vi "Lab_Temp_PID.vi"(1 "Present Value":dbl=15.0 format="%.2f", 2 "Previous Control Sum":dbl format="%.2f", 3 "Setpoint":dbl=15.0 format="%.2f") -> (0 "Dem Output":dbl format="%.2f")   [LabVIEW 2011]
uses:
  <vilib>/Analysis/NI_AALPro.lvlib
panel:
  in  "O/P deadband":dbl=0.5 format="%.2f"
  in  "Kp Deadband":dbl format="%.2f"
  in  "Derivative History":i32=20
  out "deadbanded error":dbl format="%.2f"
  in  "P":bool=TRUE
  in  "D":bool=TRUE
  in  "I":bool=TRUE
  out "Waveform Chart":T1(graph)
  in  "Manual Demand":dbl min=0.0 max=100.0 format="%.2f"
  in  "Manual Override":bool
  out "Control Sum":dbl format="%.2f"
  out "Derivative Term":dbl format="%.2f"
  out "Integral Term":dbl format="%.2f"
  out "error differential":dbl format="%.5f"
  out "error integral":dbl format="%.2f"
  out "Proportional Term":dbl format="%.2f"
  in  "Kd":dbl=50.0 format="%.2f"
  in  "Ki":dbl=40.0 format="%.2f"
  in  "Kp":dbl=30.0 format="%.2f"
  out "error":dbl format="%.2f"
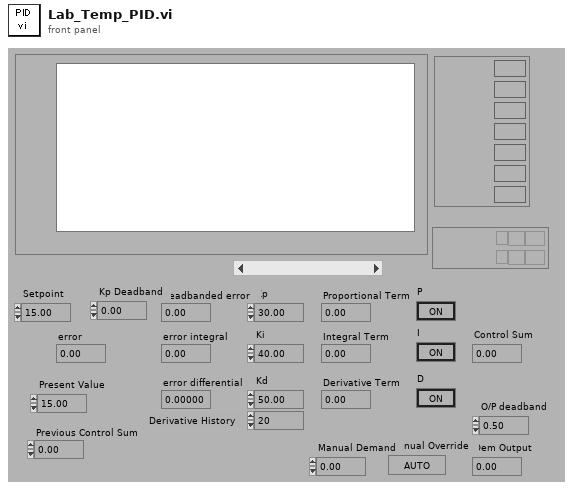
[diagram p1: front panel]
types:
  T1 = cluster{"Setpoint":dbl, "Present Value":dbl, "Proportional Term":dbl, "Integral Term":dbl, "Derivative Term":dbl, "Control Sum":dbl, "Dem Output":dbl}
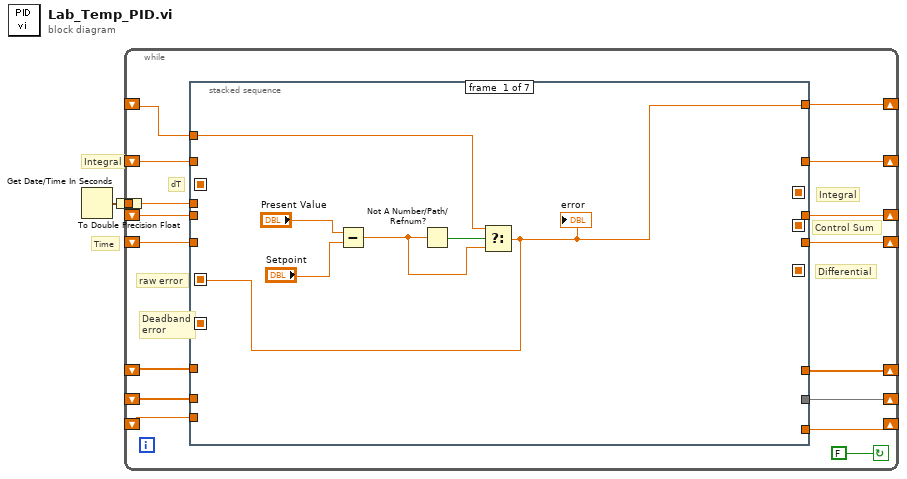
[diagram p0: block diagram]
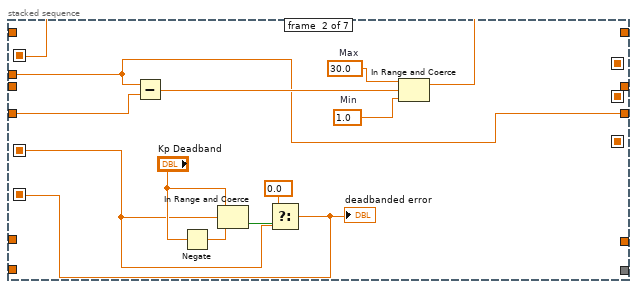
[diagram p2: hidden frame]
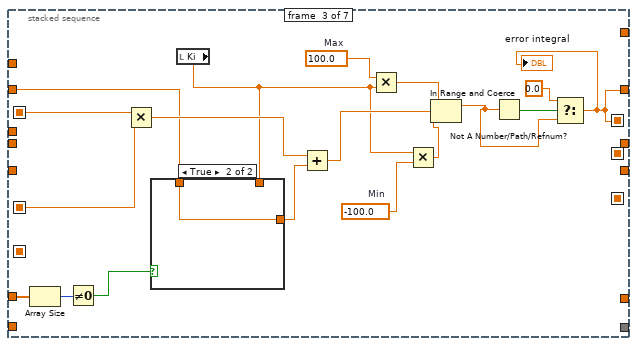
[diagram p3: hidden frame]
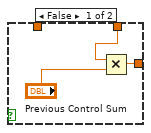
[diagram p4: hidden frame]
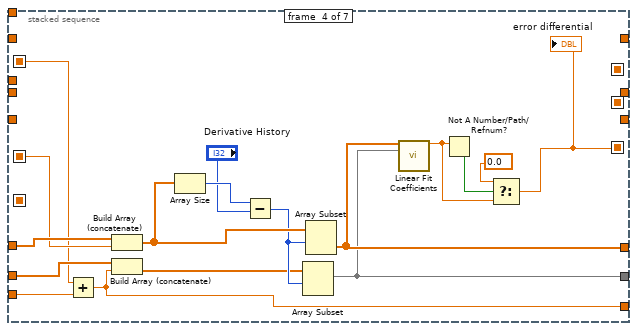
[diagram p5: hidden frame]
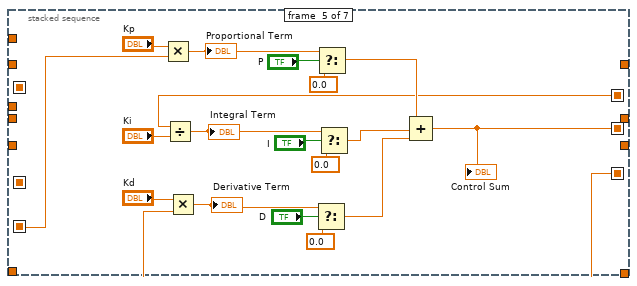
[diagram p6: hidden frame]
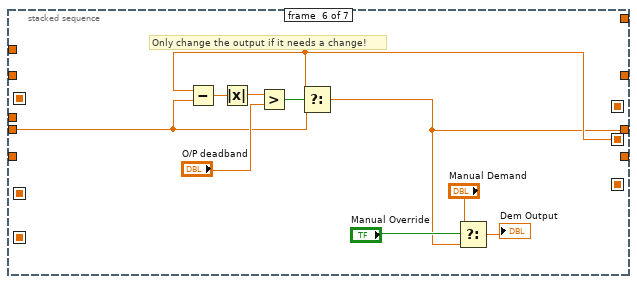
[diagram p7: hidden frame]
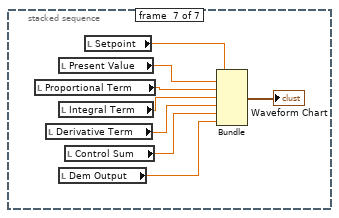
[diagram p8: hidden frame]
diagram:
  # "Integral"
  # "Time"
  n1 = Get Date/Time In Seconds() -> (seconds since 1Jan1904=w1:timestamp)
  n2 = To Double Precision Float(number=w1) -> (double precision float=w2:dbl)
  n3 = while {
    shift-left: _ -> [w5]
    shift-right: [w4] -> _
    shift-left: _ -> [w7]
    shift-right: [w6] -> _
    shift-left: _ -> [w9]
    shift-right: [w8] -> _
    tunnel: w2 -> [w14]
    shift-left: _ -> [w11]
    shift-right: [w10] -> _
    shift-left: _ -> [w13]
    shift-right: [w12] -> _
    shift-left: _ -> [w15]
    shift-right: [w16] -> _
    shift-left: _ -> [w18]
    shift-right: [w17] -> _
    stop <- FALSE continue-if-true
    # "Control Sum"
    # "raw error"
    # "Differential"
    # "Integral"
    # "Deadband\nerror"
    # "dT"
    n4 = stacked-sequence {
      seq-local: [_ w25 _ _ _ _ _] -> [_ _ w54 w61 _ _ _]
      seq-local: [_ w34 _ _ _ _ _] -> [_ _ _ _ w79 _ _]
      seq-local: [_ _ _ w66 _ _ _] -> [_ _ _ _ w78 _ _]
      seq-local: [_ _ w40 _ _ _ _] -> [_ _ _ _ w77 _ _]
      seq-local: [w20 _ _ _ _ _ _] -> [_ w26 w50 w67 _ _ _]
      seq-local: [_ _ _ _ w82 _ _] -> [_ _ _ _ _ w98 _]
      tunnel: w18 -> [_ w31 _ _ _ _ _]
      tunnel: [_ w29 _ _ _ _ _] -> w17
      tunnel: [_ _ w40 _ _ _ _] -> w16
      tunnel: w15 -> [_ _ w44 _ _ _ _]
      tunnel: w14 -> [_ w29 _ _ _ _ _]
      tunnel: w13 -> [_ _ w49 w75 _ _ _]
      tunnel: [_ _ _ w68 _ _ _] -> w12
      tunnel: w11 -> [_ _ _ w74 _ _ _]
      tunnel: [_ _ _ w65 _ _ _] -> w10
      tunnel: w9 -> [_ _ _ _ _ w96 _]
      tunnel: [_ _ _ _ _ w95 _] -> w8
      tunnel: w7 -> [_ _ _ w60 _ _ _]
      tunnel: [_ _ _ w59 _ _ _] -> w6
      tunnel: w5 -> [w21 _ _ _ _ _ _]
      tunnel: [w20 _ _ _ _ _ _] -> w4
      frame #0 {
        n5 = Subtract(x="Present Value", y="Setpoint") -> (x-y=w19:dbl)
        n6 = Not A Number/Path/Refnum?(number/path/refnum=w19) -> (NaN/Path/Refnum?=w22:bool)
        n7 = Select(t=w21, s=w22, f=w19) -> (s? t:f=w20:dbl)
        "error" <- w20
      }
      frame #1 {
        w32 = 1.0  # Min
        w33 = 30.0  # Max
        n8 = Subtract(x=w29, y=w31) -> (x-y=w30:dbl)
        n9 = Negate(x="Kp Deadband") -> (-x=w28:dbl)
        n10 = In Range and Coerce(upper limit="Kp Deadband", x=w26, lower limit=w28) -> (In Range?=w35:bool)  [unwired: 1 out]
        n11 = Select(t=0.0, s=w35, f=w26) -> (s? t:f=w34:dbl)
        "deadbanded error" <- w34
        n12 = In Range and Coerce(upper limit=w33, x=w30, lower limit=w32) -> (coerced(x)=w25:dbl)  [unwired: 1 out]
      }
      frame #2 {
        w39 = -100.0  # Min
        w53 = 100.0  # Max
        n13 = Array Size(array=w49) -> (size(s)=w48:i32)
        n14 = Not Equal To 0?(x=w48) -> (x != 0?=w46:bool)
        n15 = Multiply(x=w54, y=w50) -> (x*y=w47:dbl)
        n16 = local read "Ki"() -> (w37:dbl)
        n17 = case shown="True" w46 {
          tunnel: [w55 w58] -> w45
          tunnel: w44 -> [_ w58]
          tunnel: w37 -> [w57 _]
          frame False {
            n18 = Multiply(x=w57, y="Previous Control Sum") -> (x*y=w55:dbl)
          }
          frame True {
          }
        }
        n19 = Add(x=w47, y=w45) -> (x+y=w51:dbl)
        n20 = Multiply(x=w53, y=w37) -> (x*y=w52:dbl)
        n21 = Multiply(x=w37, y=w39) -> (x*y=w38:dbl)
        n22 = In Range and Coerce(upper limit=w52, x=w51, lower limit=w38) -> (coerced(x)=w42:dbl)  [unwired: 1 out]
        n23 = Not A Number/Path/Refnum?(number/path/refnum=w42) -> (NaN/Path/Refnum?=w43:bool)
        n24 = Select(t=0.0, s=w43, f=w42) -> (s? t:f=w40:dbl)
        "error integral" <- w40
      }
      frame #3 {
        n25 = Add(x=w61, y=w60) -> (x+y=w59:dbl)
        n26 = Build Array (concatenate)(w75, w67) -> (w71:dbl[])
        n27 = Build Array (concatenate)(w74, w59) -> (w69:dbl[])
        n28 = Array Size(array=w71) -> (size(s)=w73:i32)
        n29 = Subtract(x=w73, y="Derivative History") -> (x-y=w70:i32)
        n30 = Array Subset(array=w69, index=w70) -> (w65:dbl[])  [unwired: 1 in]
        n31 = Array Subset(array=w71, index=w70) -> (w68:dbl[])  [unwired: 1 in]
        n32 = call <vilib>:"Linear Fit Coefficients.vi"("Y"=w68, "X"=w65) -> ("slope"=w62:dbl)  [unwired: 3 in, 10 out]
        n33 = Not A Number/Path/Refnum?(number/path/refnum=w62) -> (NaN/Path/Refnum?=w64:bool)
        n34 = Select(t=0.0 ("f"), s=w64, f=w62) -> (s? t:f=w66:dbl)
        "error differential" <- w66
      }
      frame #4 {
        n35 = Multiply(x="Kp", y=w79) -> (x*y=w92:dbl)
        "Proportional Term" <- w92
        n36 = Divide(x=w77, y="Ki") -> (x/y=w83:dbl)
        "Integral Term" <- w83
        n37 = Multiply(x="Kd", y=w78) -> (x*y=w84:dbl)
        "Derivative Term" <- w84
        n38 = Select(t=w84, s="D", f=0.0) -> (s? t:f=w86:dbl)
        n39 = Select(t=w92, s="P", f=0.0) -> (s? t:f=w93:dbl)
        n40 = Select(t=w83, s="I", f=0.0) -> (s? t:f=w85:dbl)
        n41 = Compound Arithmetic op=ADD(w93, w85, w86) -> (w82:dbl)
        "Control Sum" <- w82
      }
      frame #5 {
        # "Only change the output if it needs a change!"
        n42 = Subtract(x=w98, y=w96) -> (x-y=w101:dbl)
        n43 = Absolute Value(x=w101) -> (abs(x)=w100:dbl)
        n44 = Greater?(x=w100, y="O/P deadband") -> (0:w99:bool)
        n45 = Select(t=w98, s=w99, f=w96) -> (s? t:f=w95:dbl)
        n46 = Select(t="Manual Demand", s="Manual Override", f=w95) -> (s? t:f=→"Dem Output":dbl)
      }
      frame #6 {
        n47 = local read "Proportional Term"() -> (w108:dbl)
        n48 = local read "Derivative Term"() -> (w110:dbl)
        n49 = local read "Present Value"() -> (w107:dbl)
        n50 = local read "Integral Term"() -> (w109:dbl)
        n51 = local read "Dem Output"() -> (w112:dbl)
        n52 = local read "Control Sum"() -> (w111:dbl)
        n53 = local read "Setpoint"() -> (w106:dbl)
        n54 = Bundle("Setpoint"=w106, "Present Value"=w107, "Proportional Term"=w108, "Integral Term"=w109, "Derivative Term"=w110, "Control Sum"=w111, "Dem Output"=w112) -> (→"Waveform Chart":T1)  [unwired: 1 out]
      }
    }
  }
